vi "Wave2D_Init Data_BC_Impl.vi"(9 "delta":dbl, 10 "k":dbl, 11 "Boundary Condition":cluster{"type":T1, "Value":dbl[][]} {"type" items=["Dirichlet", "Neumann"]}) -> (3 "BC":cluster{"type":T1, "Value":dbl[][]} {"type" items=["Dirichlet", "Neumann"]})   [LabVIEW 2020, in "NI_PDE.lvlib"]
uses:
  <vilib>/gmath/NI_PDE.lvlib
  <vilib>/gmath/pde.llb/Common/PDE_BC Type.ctl
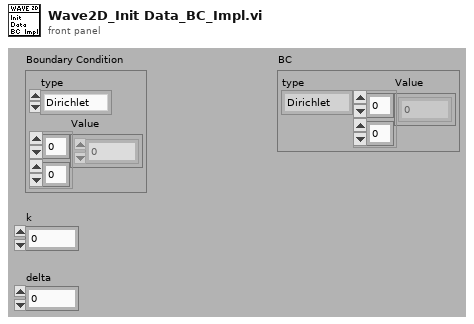
[diagram p1: front panel]
types:
  T1 = typedef "NI_PDE.lvlib/PDE_BC Type.ctl" = i32
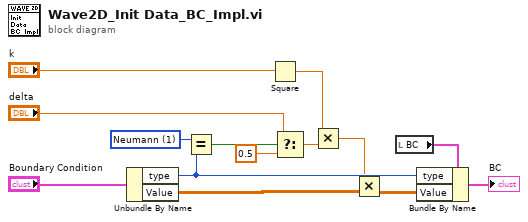
[diagram p0: block diagram]
diagram:
  w10 = T1 1 items=["Dirichlet", "Neumann"] ("x")
  n1 = Unbundle By Name("Boundary Condition") -> ("type"=w11:T1, "Value"=w1:dbl[][])
  n2 = Equal?(x=w10, y=w11) -> (x = y?=w9:bool)
  n3 = Square(x="k") -> (x^2=w4:dbl)
  n4 = Select(t="delta", s=w9, f=0.5) -> (s? t:f=w6:dbl)
  n5 = Multiply(x=w4, y=w6) -> (x*y=w3:dbl)
  n6 = Multiply(x=w3, y=w1) -> (x*y=w2:dbl[][])
  n7 = local read "BC"() -> (w13:cluster{"type":T1, "Value":dbl[][]})
  n8 = Bundle By Name(cluster=w13, "type"=w11, "Value"=w2) -> (→"BC":cluster{"type":T1, "Value":dbl[][]})
